vi "Slot Error.vi"(7 "FPGA Ref Out":T1, 8 "error in":errorcluster, 9 "timeout":u32, 10 "Start Time":u32, 11 "Previous Time":u32) -> (0 "error out":errorcluster, 1 "Slot Time":u32, 2 "Current Time":u32, 3 "Interation Duration":u32)   [LabVIEW 2021]
uses:
  Controls/FPGA Ref.ctl
  <vilib>/Utility/error.llb/Error Cluster From Error Code.vi
  <vilib>/rvi/errors/niLvFpgaAdjustHostInterfaceError.vi
  Global Variables/RT GV.vi
  <vilib>/rvi/interface/nirviReadWriteControl/nirviReadWriteControl.xnode
  <vilib>/ErrorRing/Error Ring.xnode
  NiFpgaLv.dll
  <vilib>/rvi/interface/Simulation/niFpgaSimulationCallBeginRW.vi
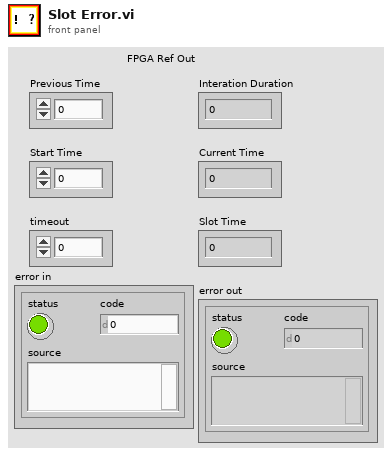
[diagram p1: front panel]
types:
  T1 = typedef "FPGA Ref.ctl" = refnum<k20>
  T2 = cluster{"Machine_ON":bool, "E_stop ":bool, "SW_Pressure":bool, "SW_Start ":bool, "SW_Reset":bool, "SW_Stop":bool, "SW_Door":bool, "Buffer 1":bool, "Buffer 2":bool, "RS_Index_Stopper _Rear":bool, "RS_Singling_Rear":bool, "PES_Index_Pallet_Sensor":bool, "PES_Index_Output_Part Sensor":bool, "Buffer 3":bool, "SW_Cutting_Station_Door":bool, "ICS_BF_Pump_CNVR_Full_1":bool, "ICS_BF_Pump_CNVR_Full_2":bool, "ICS_BF_Pump_CNVR_Full_3":bool, "ICS_BF_Pump_CNVR_Full_4":bool, "PES_PC_Pump Presence_1":bool, "PES_PC_Pump Presence_2":bool, "PES_PC_Pump Presence_3":bool, "PES_PC_Pump Presence_4":bool, "RS_Pick_Place_Vertical":bool, "Buffer 4":bool, "PES_TF_Low_Level":bool, "RS_Cutting_Rear 1":bool, "RS_Cutting_Rear 2":bool, "RS_Cutting_Rear 3":bool, "RS_Cutting_Rear 4":bool, "RS_Cutting_Forward_Rear":bool, "Buffer 10":bool}
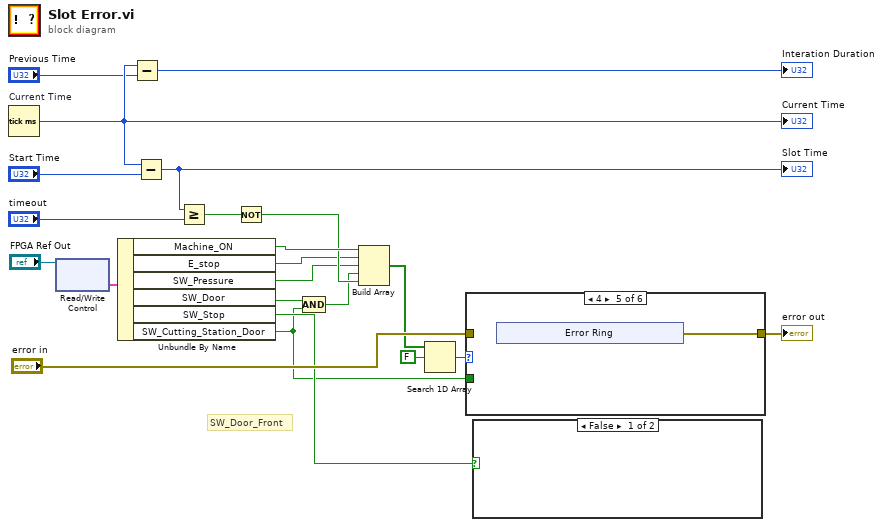
[diagram p0: block diagram]
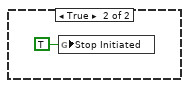
[diagram p2: hidden frame]
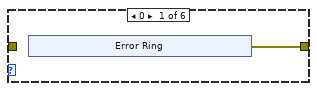
[diagram p3: hidden frame]
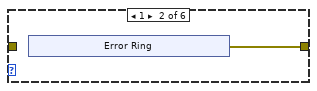
[diagram p4: hidden frame]
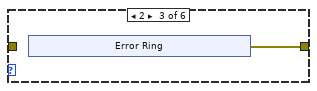
[diagram p5: hidden frame]
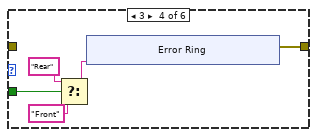
[diagram p6: hidden frame]
diagram:
  # "SW_Door_Front"
  n1 = Tick Count (ms) "Current Time"() -> (millisecond timer value=w19:u32)
  "Current Time" <- w19
  n2 = xnode "Read/Write Control"("FPGA VI Reference In"="FPGA Ref Out") -> ("DI 1"=w12:T2)  [unwired: 1 in, 2 out]
  n3 = Unbundle By Name(w12) -> ("Machine_ON"=w10:bool, "E_stop"=w5:bool, "SW_Pressure"=w4:bool, "SW_Door"=w3:bool, "SW_Stop"=w6:bool, "SW_Cutting_Station_Door"=w1:bool)
  n4 = Subtract(x=w19, y="Previous Time") -> (x-y=→"Interation Duration":u32)
  n5 = Subtract(x=w19, y="Start Time") -> (x-y=w21:u32)
  "Slot Time" <- w21
  n6 = Greater Or Equal?(x=w21, y="timeout") -> (x >= y?=w9:bool)
  n7 = Not(x=w9) -> (.not. x?=w8:bool)
  n8 = Compound Arithmetic op=AND(w3, w1) -> (w2:bool)
  n9 = Build Array(w10, w5, w4, w2, w8) -> (w7:bool[])
  n10 = Search 1D Array(1D array=w7, element=FALSE) -> (index of element=w15:i32)  [unwired: 1 in]
  n11 = case shown="4" w15 {
    tunnel: [w23 w25 w27 w33 w39 w41] -> w14
    tunnel: "error in" -> [_ _ _ _ _ w41]
    tunnel: w1 -> [_ _ _ w32 _ _]
    frame 0 {
      n12 = xnode "Error Ring"() -> ("error out"=w23:errorcluster)
    }
    frame 1 {
      n13 = xnode "Error Ring"() -> ("error out"=w25:errorcluster)
    }
    frame 2 {
      n14 = xnode "Error Ring"() -> ("error out"=w27:errorcluster)
    }
    frame 3 {
      n15 = Select(t="Rear", s=w32, f="Front") -> (s? t:f=w30:string)
      n16 = xnode "Error Ring"("parameter 0"=w30) -> ("error out"=w33:errorcluster)
    }
    frame 4 {
      n17 = xnode "Error Ring"() -> ("error out"=w39:errorcluster)
    }
    frame Default {
    }
  }
  "error out" <- w14
  n18 = case shown="False" w6 {
    frame False {
    }
    frame True {
      n19 = global write "RT GV.vi" "Stop Initiated"(TRUE ("Stop Initiated")) -> ()
    }
  }
